vi "Clear Termination Char Warning.vi"(8 "error in (no error)":errorcluster) -> (0 "error out":errorcluster)   [LabVIEW 2011, in "Magna PSU.lvlib"]
uses:
  Magna PSU.lvlib
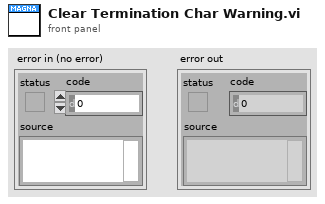
[diagram p1: front panel]
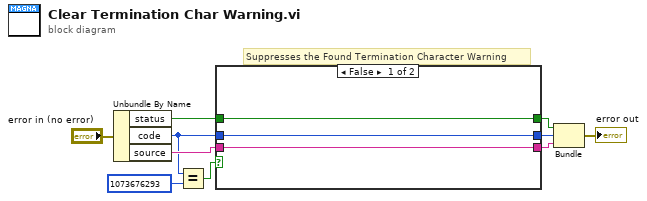
[diagram p0: block diagram]
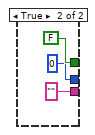
[diagram p2: hidden frame]
diagram:
  # "Suppresses the Found Termination Character Warning"
  n1 = Unbundle By Name("error in (no error)") -> ("status"=w1:bool, "code"=w4:i32, "source"=w5:string)
  n2 = Equal?(x=w4, y=1073676293) -> (x = y?=w2:bool)
  n3 = case shown="False" w2 {
    tunnel: w1 -> [w13 _]
    tunnel: w4 -> [w12 _]
    tunnel: [w13 FALSE] -> w6
    tunnel: w5 -> [w11 _]
    tunnel: [w12 0] -> w8
    tunnel: [w11 ""] -> w7
    frame False {
    }
    frame True {
    }
  }
  n4 = Bundle("status"=w6, "code"=w8, "source"=w7) -> (→"error out":errorcluster)  [unwired: 1 in]
